vi "Get PID Drive Straight Gains.vi"(11 "drive in":refnum<class "drive.lvclass">) -> (2 "PID Drive Straight Gains":T1, 3 "drive out":refnum<class "drive.lvclass">)   [LabVIEW 2015, in "drive.lvclass"]
uses:
  drive.lvclass
  drive.lvclass/drive.ctl
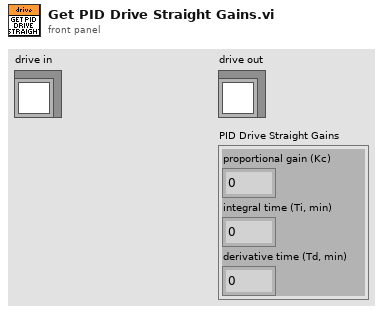
[diagram p1: front panel]
types:
  T1 = cluster{"proportional gain (Kc)":dbl, "integral time (Ti, min)":dbl, "derivative time (Td, min)":dbl}
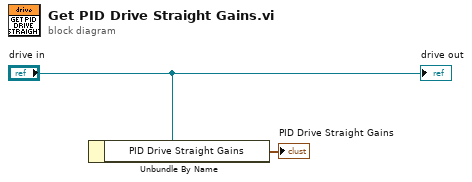
[diagram p0: block diagram]
diagram:
  n1 = Unbundle By Name("drive in") -> ("PID Drive Straight Gains"=→"PID Drive Straight Gains":T1)
  "drive out" <- "drive in"
